vi "p45_1_mean value.vi"() -> ()   [LabVIEW 2013]
uses:
  <vilib>/Analysis/baseanly.llb/Mean (DBL).vi
  <vilib>/Analysis/NI_AALBase.lvlib
panel:
  out "mean by max":dbl
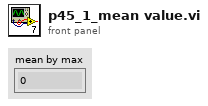
[diagram p1: front panel]
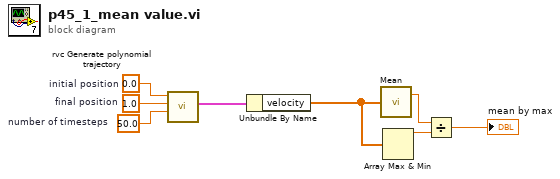
[diagram p0: block diagram]
diagram:
  w5 = 50.0  # number of timesteps
  w4 = 1.0  # final position
  w3 = 0.0  # initial position
  n1 = call "rvc Generate polynomial trajectory.vi"("number of timesteps"=w5, "final position"=w4, "initial position"=w3) -> ("velocity"=w1:cluster{"time":dbl[], "velocity":dbl[]})  [unwired: 6 in, 2 out]
  n2 = Unbundle By Name "Unbundle By Name"(w1) -> ("velocity"=w2:dbl[])
  n3 = call-poly <vilib>:"Mean.vi"("X"=w2) -> ("mean"=w8:dbl)  [unwired: 1 out]
  n4 = Array Max & Min(array=w2) -> (max value=w7:dbl)  [unwired: 3 out]
  n5 = Divide(x=w8, y=w7) -> (x/y=→"mean by max":dbl)
